vi "runSnapper.vi"(8 "error in (no error)":errorcluster) -> (0 "error out":errorcluster)   [LabVIEW 2009, in "iManagement.lvlib" / "CameraManager.lvclass"]
uses:
  CameraManager.lvclass
  CameraManager.lvclass/CameraManager.ctl
  Hal/Channels/Camera/CameraController.lvclass
  Hal/Channels/Camera/CameraEventsManager/CameraEventsManger.lvclass
  Viewers/Snapper.lvclass
panel:
  in  "CameraManager.lvclass":refnum<class "CameraManager.lvclass">
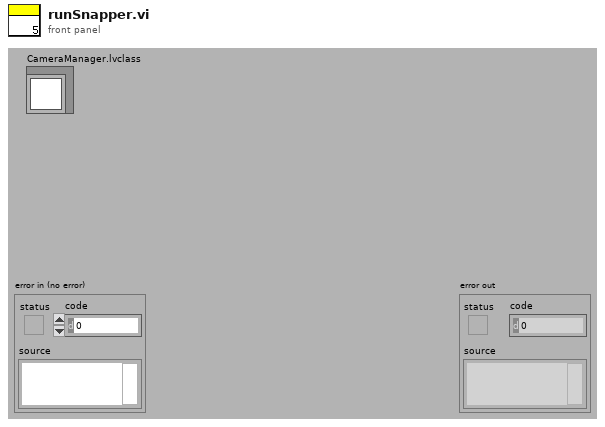
[diagram p1: front panel]
types:
  T1 = cluster{"settingsFrontEndEvents":cluster{"loadSettingsFromPath":refnum<user-event>, "lookUpElementEvent":refnum<user-event>, "saveSettings":refnum<user-event>, "loadSettings":refnum<user-event>, "close":refnum<user-event>, "replaceElement":refnum<user-event>, "findParentNodes":refnum<user-event>, "createNode":refnum<user-event>}, "settingBackEndEvents":cluster{"defaultSettingsPathRequest":refnum<user-event>, "searchResultEvent":refnum<user-event>, "settingsSaved":refnum<user-event>, "settingsLoaded":refnum<user-event>, "foundParentNode":refnum<user-event>}}
  T2 = cluster{"frontEndEvents":cluster{"snapShotEvent":refnum<user-event>, "stopShooting":refnum<user-event>, "userSnapShot":refnum<user-event>}, "backEndEvents":cluster{"picture":refnum<user-event>}}
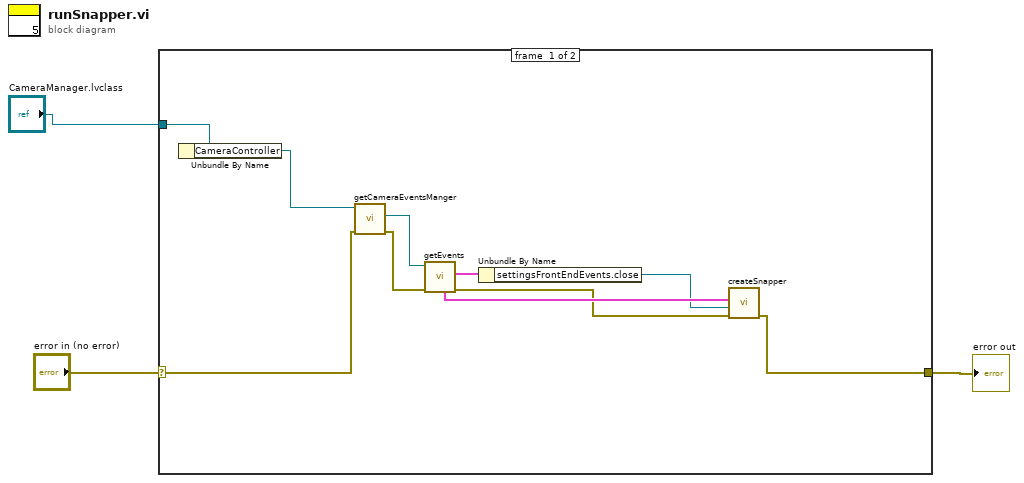
[diagram p0: block diagram]
diagram:
  n1 = case shown="No Error" "error in (no error)" {
    selector: "error in (no error)" -> [w10 w14]
    tunnel: [w6 w14] -> w2
    tunnel: "CameraManager.lvclass" -> [w5 _]
    frame #0 {
      n2 = Unbundle By Name(w5) -> ("CameraController"=w4:refnum<class "CameraController.lvclass">)
      n3 = call-dynamic "getCameraEventsManger.vi"("error in (no error)"=w10, "CameraController.lvclass in"=w4) -> ("error out"=w12:errorcluster, "Hardware:Channels.lvlib:CameraEventsManger.lvclass"=w13:refnum<class "CameraEventsManger.lvclass">)  [unwired: 7 in, 1 out]
      n4 = call-dynamic "getEvents.vi"("error in (no error)"=w12, "CameraEventsManger in"=w13) -> ("error out"=w7:errorcluster, "settingsEvents"=w11:T1, "snapperEvents"=w9:T2)  [unwired: 5 in, 2 out]
      n5 = Unbundle By Name(w11) -> ("settingsFrontEndEvents.close"=w8:refnum<user-event>)
      n6 = call "createSnapper.vi"("error in (no error)"=w7, "close"=w8, "snapperEvents"=w9) -> ("error out"=w6:errorcluster)  [unwired: 7 in, 1 out]
    }
    frame #1 {
    }
  }
  "error out" <- w2
